vi "aws.vi"() -> ()   [LabVIEW 2016]
panel:
  in  "AWS Credentials":T1={"Access Key"="AKIAIVLJ32AQWAW5XJMA", "Secret Key"="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\n+V46TU/7fiFpPcYmKK6mtiPZO7SPIgfTvZgCsNmP\n+V46TU/7fiFpPcYmKK6mtiPZO7SPIgfTvZgCsNmP\n+V46TU/7fiFpPcYmKK6mtiPZO7SPIgfTvZgCsNmP"}
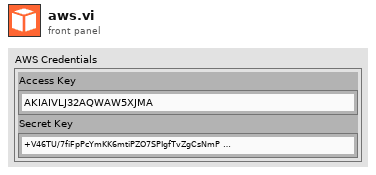
[diagram p1: front panel]
types:
  T1 = cluster{"Access Key":string, "Secret Key":string}
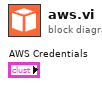
[diagram p0: block diagram]
diagram:
